vi "Lab Panel V4.84.vi"() -> ()   [LabVIEW 2013] (continued)
                            n2010 = Bundle By Name("Y"=w3276, "t0"=w3271) -> (w3268:waveform(dbl))  [unwired: 1 in]
                            n2011 = Bundle By Name("Y"=w3275, "t0"=w3271) -> (w3267:waveform(dbl))  [unwired: 1 in]
                            n2012 = Bundle By Name("Y"=w3274, "t0"=w3271) -> (w3266:waveform(dbl))  [unwired: 1 in]
                            n2013 = Bundle By Name("Y"=w3273, "t0"=w3271) -> (w3265:waveform(dbl))  [unwired: 1 in]
                            n2014 = Bundle By Name("Y"=w3272, "t0"=w3271) -> (w3264:waveform(dbl))  [unwired: 1 in]
                            n2015 = Build Array(w3270, w3269, w3268, w3267, w3266, w3265, w3264) -> (w3263:waveform(dbl)[])
                            n2016 = TDMS Write(0:w3284, 5:"TEST VALUES", 7:w3255, 9:w3263) -> (4:w3254:refnum<k34>, 6:w3253:string, 15:w3252:errorcluster)  [unwired: 2 in, 1 out]
                            n2017 = TDMS Write(0:w3254, 5:w3253, 7:"TIME", 9:w3250, 11:w3252) -> (15:w3249:errorcluster)  [unwired: 1 in, 3 out]
                            n2018 = local write "data file error"(w3249) -> ()
                          }
                        }
                      }
                    }
                  }
                }
              }
              frame #2 {
                n2019 = case shown="True" w3288 {
                  tunnel: w3292 -> [_ w3297]
                  tunnel: w3291 -> [_ w3296]
                  tunnel: w3290 -> [_ w3294]
                  tunnel: w3289 -> [_ w3293]
                  frame False {
                  }
                  frame True {
                    n2020 = local read "DISP LAB02-1"() -> (w3298:T4)
                    n2021 = local read "SIG LAB02-1"() -> (w3299:T2)
                    n2022 = local read "ON L02-1"() -> (w3295:cluster{"amps":dbl, "volts":dbl, "pf":dbl})
                    n2023 = Unbundle(w3299) -> ("AMPS"=w3305:dbl, "VOLTS"=w3303:dbl, "PF"=w3302:dbl, "Tmp Live"=w3301:dbl, "Tmp Neut"=w3304:dbl)
                    n2024 = Unbundle(w3298) -> ("CYCLE"=w3300:dbl)  [unwired: 2 out]
                    n2025 = stacked-sequence {
                      tunnel: w3305 -> [w3309 w3328]
                      tunnel: w3304 -> [_ w3327]
                      tunnel: w3303 -> [w3308 w3326]
                      tunnel: w3302 -> [w3307 w3325]
                      tunnel: w3301 -> [_ w3324]
                      tunnel: w3300 -> [_ w3323]
                      tunnel: w3297 -> [_ w3322]
                      tunnel: w3296 -> [w3310 _]
                      tunnel: w3295 -> [w3306 w3320]
                      tunnel: w3294 -> [_ w3321]
                      tunnel: w3293 -> [_ w3316]
                      frame #0 {
                        n2026 = case shown="True" w3310 {
                          tunnel: w3309 -> [_ w3315]
                          tunnel: w3308 -> [_ w3314]
                          tunnel: w3307 -> [_ w3313]
                          tunnel: w3306 -> [_ w3311]
                          frame False {
                          }
                          frame True {
                            n2027 = Bundle(cluster=w3311, "amps"=w3315, "volts"=w3314, "pf"=w3313) -> (w3312:cluster{"amps":dbl, "volts":dbl, "pf":dbl})
                            n2028 = local write "ON L02-1"(w3312) -> ()
                          }
                        }
                      }
                      frame #1 {
                        n2029 = Unbundle(w3320) -> ("amps"=w3319:dbl, "volts"=w3318:dbl, "pf"=w3317:dbl)
                        n2030 = case shown="True" w3321 {
                          tunnel: w3328 -> [_ w3360]
                          tunnel: w3327 -> [_ w3367]
                          tunnel: w3326 -> [_ _]
                          tunnel: w3325 -> [_ _]
                          tunnel: w3324 -> [_ w3366]
                          tunnel: w3323 -> [_ w3365]
                          tunnel: w3322 -> [_ w3330]
                          tunnel: w3319 -> [_ w3362]
                          tunnel: w3318 -> [_ w3361]
                          tunnel: w3317 -> [_ w3359]
                          tunnel: w3316 -> [_ w3351]
                          frame False {
                          }
                          frame True {
                            n2031 = local read "TDMS LAB02-1"() -> (w3364:refnum<k34>)
                            n2032 = Build Array(w3361) -> (w3356:dbl[])
                            n2033 = Build Array(w3359) -> (w3355:dbl[])
                            n2034 = Build Array(w3366) -> (w3354:dbl[])
                            n2035 = Build Array(w3367) -> (w3353:dbl[])
                            n2036 = Build Array(w3362) -> (w3358:dbl[])
                            n2037 = Build Array(w3360) -> (w3357:dbl[])
                            n2038 = Build Array(w3365) -> (w3352:dbl[])
                            n2039 = Build Array("AMPS ON", "AMPS OFF", "VOLTS", "PF", "TEMP Live", "TEMP Neut", "CYCLE") -> (w3335:string[])
                            n2040 = Bundle By Name("Y"=w3358, "t0"=w3351) -> (w3350:waveform(dbl))  [unwired: 1 in]
                            n2041 = Bundle By Name("Y"=w3357, "t0"=w3351) -> (w3349:waveform(dbl))  [unwired: 1 in]
                            n2042 = Bundle By Name("Y"=w3356, "t0"=w3351) -> (w3348:waveform(dbl))  [unwired: 1 in]
                            n2043 = Bundle By Name("Y"=w3355, "t0"=w3351) -> (w3347:waveform(dbl))  [unwired: 1 in]
                            n2044 = Bundle By Name("Y"=w3354, "t0"=w3351) -> (w3346:waveform(dbl))  [unwired: 1 in]
                            n2045 = Bundle By Name("Y"=w3353, "t0"=w3351) -> (w3345:waveform(dbl))  [unwired: 1 in]
                            n2046 = Bundle By Name("Y"=w3352, "t0"=w3351) -> (w3344:waveform(dbl))  [unwired: 1 in]
                            n2047 = Build Array(w3350, w3349, w3348, w3347, w3346, w3345, w3344) -> (w3343:waveform(dbl)[])
                            n2048 = TDMS Write(0:w3364, 5:"TEST VALUES", 7:w3335, 9:w3343) -> (4:w3334:refnum<k34>, 6:w3333:string, 15:w3332:errorcluster)  [unwired: 2 in, 1 out]
                            n2049 = TDMS Write(0:w3334, 5:w3333, 7:"TIME", 9:w3330, 11:w3332) -> (15:w3329:errorcluster)  [unwired: 1 in, 3 out]
                            n2050 = local write "data file error"(w3329) -> ()
                          }
                        }
                      }
                    }
                  }
                }
              }
              frame #3 {
                n2051 = case shown="True" w3368 {
                  tunnel: w3372 -> [_ w3377]
                  tunnel: w3371 -> [_ w3376]
                  tunnel: w3370 -> [_ w3374]
                  tunnel: w3369 -> [_ w3373]
                  frame False {
                  }
                  frame True {
                    n2052 = local read "DISP LAB02-2"() -> (w3378:T4)
                    n2053 = local read "SIG LAB02-2"() -> (w3379:T2)
                    n2054 = local read "ON L02-2"() -> (w3375:cluster{"amps":dbl, "volts":dbl, "pf":dbl})
                    n2055 = Unbundle(w3379) -> ("AMPS"=w3385:dbl, "VOLTS"=w3383:dbl, "PF"=w3382:dbl, "Tmp Live"=w3381:dbl, "Tmp Neut"=w3384:dbl)
                    n2056 = Unbundle(w3378) -> ("CYCLE"=w3380:dbl)  [unwired: 2 out]
                    n2057 = stacked-sequence {
                      tunnel: w3385 -> [w3389 w3408]
                      tunnel: w3384 -> [_ w3407]
                      tunnel: w3383 -> [w3388 w3406]
                      tunnel: w3382 -> [w3387 w3405]
                      tunnel: w3381 -> [_ w3404]
                      tunnel: w3380 -> [_ w3403]
                      tunnel: w3377 -> [_ w3402]
                      tunnel: w3376 -> [w3390 _]
                      tunnel: w3375 -> [w3386 w3400]
                      tunnel: w3374 -> [_ w3401]
                      tunnel: w3373 -> [_ w3396]
                      frame #0 {
                        n2058 = case shown="True" w3390 {
                          tunnel: w3389 -> [_ w3395]
                          tunnel: w3388 -> [_ w3394]
                          tunnel: w3387 -> [_ w3393]
                          tunnel: w3386 -> [_ w3391]
                          frame False {
                          }
                          frame True {
                            n2059 = Bundle(cluster=w3391, "amps"=w3395, "volts"=w3394, "pf"=w3393) -> (w3392:cluster{"amps":dbl, "volts":dbl, "pf":dbl})
                            n2060 = local write "ON L02-2"(w3392) -> ()
                          }
                        }
                      }
                      frame #1 {
                        n2061 = Unbundle(w3400) -> ("amps"=w3399:dbl, "volts"=w3398:dbl, "pf"=w3397:dbl)
                        n2062 = case shown="True" w3401 {
                          tunnel: w3408 -> [_ w3440]
                          tunnel: w3407 -> [_ w3447]
                          tunnel: w3406 -> [_ _]
                          tunnel: w3405 -> [_ _]
                          tunnel: w3404 -> [_ w3446]
                          tunnel: w3403 -> [_ w3445]
                          tunnel: w3402 -> [_ w3410]
                          tunnel: w3399 -> [_ w3442]
                          tunnel: w3398 -> [_ w3441]
                          tunnel: w3397 -> [_ w3439]
                          tunnel: w3396 -> [_ w3431]
                          frame False {
                          }
                          frame True {
                            n2063 = local read "TDMS LAB02-2"() -> (w3444:refnum<k34>)
                            n2064 = Build Array(w3441) -> (w3436:dbl[])
                            n2065 = Build Array(w3439) -> (w3435:dbl[])
                            n2066 = Build Array(w3446) -> (w3434:dbl[])
                            n2067 = Build Array(w3447) -> (w3433:dbl[])
                            n2068 = Build Array(w3442) -> (w3438:dbl[])
                            n2069 = Build Array(w3440) -> (w3437:dbl[])
                            n2070 = Build Array(w3445) -> (w3432:dbl[])
                            n2071 = Build Array("AMPS ON", "AMPS OFF", "VOLTS", "PF", "TEMP Live", "TEMP Neut", "CYCLE") -> (w3415:string[])
                            n2072 = Bundle By Name("Y"=w3438, "t0"=w3431) -> (w3430:waveform(dbl))  [unwired: 1 in]
                            n2073 = Bundle By Name("Y"=w3437, "t0"=w3431) -> (w3429:waveform(dbl))  [unwired: 1 in]
                            n2074 = Bundle By Name("Y"=w3436, "t0"=w3431) -> (w3428:waveform(dbl))  [unwired: 1 in]
                            n2075 = Bundle By Name("Y"=w3435, "t0"=w3431) -> (w3427:waveform(dbl))  [unwired: 1 in]
                            n2076 = Bundle By Name("Y"=w3434, "t0"=w3431) -> (w3426:waveform(dbl))  [unwired: 1 in]
                            n2077 = Bundle By Name("Y"=w3433, "t0"=w3431) -> (w3425:waveform(dbl))  [unwired: 1 in]
                            n2078 = Bundle By Name("Y"=w3432, "t0"=w3431) -> (w3424:waveform(dbl))  [unwired: 1 in]
                            n2079 = Build Array(w3430, w3429, w3428, w3427, w3426, w3425, w3424) -> (w3423:waveform(dbl)[])
                            n2080 = TDMS Write(0:w3444, 5:"TEST VALUES", 7:w3415, 9:w3423) -> (4:w3414:refnum<k34>, 6:w3413:string, 15:w3412:errorcluster)  [unwired: 2 in, 1 out]
                            n2081 = TDMS Write(0:w3414, 5:w3413, 7:"TIME", 9:w3410, 11:w3412) -> (15:w3409:errorcluster)  [unwired: 1 in, 3 out]
                            n2082 = local write "data file error"(w3409) -> ()
                          }
                        }
                      }
                    }
                  }
                }
              }
              frame #4 {
                n2083 = case shown="True" w3448 {
                  tunnel: w3452 -> [_ w3457]
                  tunnel: w3451 -> [_ w3456]
                  tunnel: w3450 -> [_ w3454]
                  tunnel: w3449 -> [_ w3453]
                  frame False {
                  }
                  frame True {
                    n2084 = local read "DISP LAB03-1"() -> (w3458:T4)
                    n2085 = local read "SIG LAB03-1"() -> (w3459:T2)
                    n2086 = local read "ON L03-1"() -> (w3455:cluster{"amps":dbl, "volts":dbl, "pf":dbl})
                    n2087 = Unbundle(w3459) -> ("AMPS"=w3465:dbl, "VOLTS"=w3463:dbl, "PF"=w3462:dbl, "Tmp Live"=w3461:dbl, "Tmp Neut"=w3464:dbl)
                    n2088 = Unbundle(w3458) -> ("CYCLE"=w3460:dbl)  [unwired: 2 out]
                    n2089 = stacked-sequence {
                      tunnel: w3465 -> [w3469 w3488]
                      tunnel: w3464 -> [_ w3487]
                      tunnel: w3463 -> [w3468 w3486]
                      tunnel: w3462 -> [w3467 w3485]
                      tunnel: w3461 -> [_ w3484]
                      tunnel: w3460 -> [_ w3483]
                      tunnel: w3457 -> [_ w3482]
                      tunnel: w3456 -> [w3470 _]
                      tunnel: w3455 -> [w3466 w3480]
                      tunnel: w3454 -> [_ w3481]
                      tunnel: w3453 -> [_ w3476]
                      frame #0 {
                        n2090 = case shown="True" w3470 {
                          tunnel: w3469 -> [_ w3475]
                          tunnel: w3468 -> [_ w3474]
                          tunnel: w3467 -> [_ w3473]
                          tunnel: w3466 -> [_ w3471]
                          frame False {
                          }
                          frame True {
                            n2091 = Bundle(cluster=w3471, "amps"=w3475, "volts"=w3474, "pf"=w3473) -> (w3472:cluster{"amps":dbl, "volts":dbl, "pf":dbl})
                            n2092 = local write "ON L03-1"(w3472) -> ()
                          }
                        }
                      }
                      frame #1 {
                        n2093 = Unbundle(w3480) -> ("amps"=w3479:dbl, "volts"=w3478:dbl, "pf"=w3477:dbl)
                        n2094 = case shown="True" w3481 {
                          tunnel: w3488 -> [_ w3520]
                          tunnel: w3487 -> [_ w3527]
                          tunnel: w3486 -> [_ _]
                          tunnel: w3485 -> [_ _]
                          tunnel: w3484 -> [_ w3526]
                          tunnel: w3483 -> [_ w3525]
                          tunnel: w3482 -> [_ w3490]
                          tunnel: w3479 -> [_ w3522]
                          tunnel: w3478 -> [_ w3521]
                          tunnel: w3477 -> [_ w3519]
                          tunnel: w3476 -> [_ w3511]
                          frame False {
                          }
                          frame True {
                            n2095 = local read "TDMS LAB03-1"() -> (w3524:refnum<k34>)
                            n2096 = Build Array(w3521) -> (w3516:dbl[])
                            n2097 = Build Array(w3519) -> (w3515:dbl[])
                            n2098 = Build Array(w3526) -> (w3514:dbl[])
                            n2099 = Build Array(w3527) -> (w3513:dbl[])
                            n2100 = Build Array(w3522) -> (w3518:dbl[])
                            n2101 = Build Array(w3520) -> (w3517:dbl[])
                            n2102 = Build Array(w3525) -> (w3512:dbl[])
                            n2103 = Build Array("AMPS ON", "AMPS OFF", "VOLTS", "PF", "TEMP Live", "TEMP Neut", "CYCLE") -> (w3495:string[])
                            n2104 = Bundle By Name("Y"=w3518, "t0"=w3511) -> (w3510:waveform(dbl))  [unwired: 1 in]
                            n2105 = Bundle By Name("Y"=w3517, "t0"=w3511) -> (w3509:waveform(dbl))  [unwired: 1 in]
                            n2106 = Bundle By Name("Y"=w3516, "t0"=w3511) -> (w3508:waveform(dbl))  [unwired: 1 in]
                            n2107 = Bundle By Name("Y"=w3515, "t0"=w3511) -> (w3507:waveform(dbl))  [unwired: 1 in]
                            n2108 = Bundle By Name("Y"=w3514, "t0"=w3511) -> (w3506:waveform(dbl))  [unwired: 1 in]
                            n2109 = Bundle By Name("Y"=w3513, "t0"=w3511) -> (w3505:waveform(dbl))  [unwired: 1 in]
                            n2110 = Bundle By Name("Y"=w3512, "t0"=w3511) -> (w3504:waveform(dbl))  [unwired: 1 in]
                            n2111 = Build Array(w3510, w3509, w3508, w3507, w3506, w3505, w3504) -> (w3503:waveform(dbl)[])
                            n2112 = TDMS Write(0:w3524, 5:"TEST VALUES", 7:w3495, 9:w3503) -> (4:w3494:refnum<k34>, 6:w3493:string, 15:w3492:errorcluster)  [unwired: 2 in, 1 out]
                            n2113 = TDMS Write(0:w3494, 5:w3493, 7:"TIME", 9:w3490, 11:w3492) -> (15:w3489:errorcluster)  [unwired: 1 in, 3 out]
                            n2114 = local write "data file error"(w3489) -> ()
                          }
                        }
                      }
                    }
                  }
                }
              }
              frame #5 {
                n2115 = case shown="True" w3528 {
                  tunnel: w3532 -> [_ w3537]
                  tunnel: w3531 -> [_ w3536]
                  tunnel: w3530 -> [_ w3534]
                  tunnel: w3529 -> [_ w3533]
                  frame False {
                  }
                  frame True {
                    n2116 = local read "DISP LAB03-2"() -> (w3538:T4)
                    n2117 = local read "SIG LAB03-2"() -> (w3539:T2)
                    n2118 = local read "ON L03-2"() -> (w3535:cluster{"amps":dbl, "volts":dbl, "pf":dbl})
                    n2119 = Unbundle(w3539) -> ("AMPS"=w3545:dbl, "VOLTS"=w3543:dbl, "PF"=w3542:dbl, "Tmp Live"=w3541:dbl, "Tmp Neut"=w3544:dbl)
                    n2120 = Unbundle(w3538) -> ("CYCLE"=w3540:dbl)  [unwired: 2 out]
                    n2121 = stacked-sequence {
                      tunnel: w3545 -> [w3549 w3568]
                      tunnel: w3544 -> [_ w3567]
                      tunnel: w3543 -> [w3548 w3566]
                      tunnel: w3542 -> [w3547 w3565]
                      tunnel: w3541 -> [_ w3564]
                      tunnel: w3540 -> [_ w3563]
                      tunnel: w3537 -> [_ w3562]
                      tunnel: w3536 -> [w3550 _]
                      tunnel: w3535 -> [w3546 w3560]
                      tunnel: w3534 -> [_ w3561]
                      tunnel: w3533 -> [_ w3556]
                      frame #0 {
                        n2122 = case shown="True" w3550 {
                          tunnel: w3549 -> [_ w3555]
                          tunnel: w3548 -> [_ w3554]
                          tunnel: w3547 -> [_ w3553]
                          tunnel: w3546 -> [_ w3551]
                          frame False {
                          }
                          frame True {
                            n2123 = Bundle(cluster=w3551, "amps"=w3555, "volts"=w3554, "pf"=w3553) -> (w3552:cluster{"amps":dbl, "volts":dbl, "pf":dbl})
                            n2124 = local write "ON L03-2"(w3552) -> ()
                          }
                        }
                      }
                      frame #1 {
                        n2125 = Unbundle(w3560) -> ("amps"=w3559:dbl, "volts"=w3558:dbl, "pf"=w3557:dbl)
                        n2126 = case shown="True" w3561 {
                          tunnel: w3568 -> [_ w3600]
                          tunnel: w3567 -> [_ w3607]
                          tunnel: w3566 -> [_ _]
                          tunnel: w3565 -> [_ _]
                          tunnel: w3564 -> [_ w3606]
                          tunnel: w3563 -> [_ w3605]
                          tunnel: w3562 -> [_ w3570]
                          tunnel: w3559 -> [_ w3602]
                          tunnel: w3558 -> [_ w3601]
                          tunnel: w3557 -> [_ w3599]
                          tunnel: w3556 -> [_ w3591]
                          frame False {
                          }
                          frame True {
                            n2127 = local read "TDMS LAB03-2"() -> (w3604:refnum<k34>)
                            n2128 = Build Array(w3601) -> (w3596:dbl[])
                            n2129 = Build Array(w3599) -> (w3595:dbl[])
                            n2130 = Build Array(w3606) -> (w3594:dbl[])
                            n2131 = Build Array(w3607) -> (w3593:dbl[])
                            n2132 = Build Array(w3602) -> (w3598:dbl[])
                            n2133 = Build Array(w3600) -> (w3597:dbl[])
                            n2134 = Build Array(w3605) -> (w3592:dbl[])
                            n2135 = Build Array("AMPS ON", "AMPS OFF", "VOLTS", "PF", "TEMP Live", "TEMP Neut", "CYCLE") -> (w3575:string[])
                            n2136 = Bundle By Name("Y"=w3598, "t0"=w3591) -> (w3590:waveform(dbl))  [unwired: 1 in]
                            n2137 = Bundle By Name("Y"=w3597, "t0"=w3591) -> (w3589:waveform(dbl))  [unwired: 1 in]
                            n2138 = Bundle By Name("Y"=w3596, "t0"=w3591) -> (w3588:waveform(dbl))  [unwired: 1 in]
                            n2139 = Bundle By Name("Y"=w3595, "t0"=w3591) -> (w3587:waveform(dbl))  [unwired: 1 in]
                            n2140 = Bundle By Name("Y"=w3594, "t0"=w3591) -> (w3586:waveform(dbl))  [unwired: 1 in]
                            n2141 = Bundle By Name("Y"=w3593, "t0"=w3591) -> (w3585:waveform(dbl))  [unwired: 1 in]
                            n2142 = Bundle By Name("Y"=w3592, "t0"=w3591) -> (w3584:waveform(dbl))  [unwired: 1 in]
                            n2143 = Build Array(w3590, w3589, w3588, w3587, w3586, w3585, w3584) -> (w3583:waveform(dbl)[])
                            n2144 = TDMS Write(0:w3604, 5:"TEST VALUES", 7:w3575, 9:w3583) -> (4:w3574:refnum<k34>, 6:w3573:string, 15:w3572:errorcluster)  [unwired: 2 in, 1 out]
                            n2145 = TDMS Write(0:w3574, 5:w3573, 7:"TIME", 9:w3570, 11:w3572) -> (15:w3569:errorcluster)  [unwired: 1 in, 3 out]
                            n2146 = local write "data file error"(w3569) -> ()
                          }
                        }
                      }
                    }
                  }
                }
              }
              frame #6 {
                n2147 = case shown="True" w3608 {
                  tunnel: w3612 -> [_ w3617]
                  tunnel: w3611 -> [_ w3616]
                  tunnel: w3610 -> [_ w3614]
                  tunnel: w3609 -> [_ w3613]
                  frame False {
                  }
                  frame True {
                    n2148 = local read "DISP LAB04-1"() -> (w3618:T4)
                    n2149 = local read "SIG LAB04-1"() -> (w3619:T2)
                    n2150 = local read "ON L04-1"() -> (w3615:cluster{"amps":dbl, "volts":dbl, "pf":dbl})
                    n2151 = Unbundle(w3619) -> ("AMPS"=w3625:dbl, "VOLTS"=w3623:dbl, "PF"=w3622:dbl, "Tmp Live"=w3621:dbl, "Tmp Neut"=w3624:dbl)
                    n2152 = Unbundle(w3618) -> ("CYCLE"=w3620:dbl)  [unwired: 2 out]
                    n2153 = stacked-sequence {
                      tunnel: w3625 -> [w3629 w3648]
                      tunnel: w3624 -> [_ w3647]
                      tunnel: w3623 -> [w3628 w3646]
                      tunnel: w3622 -> [w3627 w3645]
                      tunnel: w3621 -> [_ w3644]
                      tunnel: w3620 -> [_ w3643]
                      tunnel: w3617 -> [_ w3642]
                      tunnel: w3616 -> [w3630 _]
                      tunnel: w3615 -> [w3626 w3640]
                      tunnel: w3614 -> [_ w3641]
                      tunnel: w3613 -> [_ w3636]
                      frame #0 {
                        n2154 = case shown="True" w3630 {
                          tunnel: w3629 -> [_ w3635]
                          tunnel: w3628 -> [_ w3634]
                          tunnel: w3627 -> [_ w3633]
                          tunnel: w3626 -> [_ w3631]
                          frame False {
                          }
                          frame True {
                            n2155 = Bundle(cluster=w3631, "amps"=w3635, "volts"=w3634, "pf"=w3633) -> (w3632:cluster{"amps":dbl, "volts":dbl, "pf":dbl})
                            n2156 = local write "ON L04-1"(w3632) -> ()
                          }
                        }
                      }
                      frame #1 {
                        n2157 = Unbundle(w3640) -> ("amps"=w3639:dbl, "volts"=w3638:dbl, "pf"=w3637:dbl)
                        n2158 = case shown="True" w3641 {
                          tunnel: w3648 -> [_ w3680]
                          tunnel: w3647 -> [_ w3687]
                          tunnel: w3646 -> [_ _]
                          tunnel: w3645 -> [_ _]
                          tunnel: w3644 -> [_ w3686]
                          tunnel: w3643 -> [_ w3685]
                          tunnel: w3642 -> [_ w3650]
                          tunnel: w3639 -> [_ w3682]
                          tunnel: w3638 -> [_ w3681]
                          tunnel: w3637 -> [_ w3679]
                          tunnel: w3636 -> [_ w3671]
                          frame False {
                          }
                          frame True {
                            n2159 = local read "TDMS LAB04-1"() -> (w3684:refnum<k34>)
                            n2160 = Build Array(w3681) -> (w3676:dbl[])
                            n2161 = Build Array(w3679) -> (w3675:dbl[])
                            n2162 = Build Array(w3686) -> (w3674:dbl[])
                            n2163 = Build Array(w3687) -> (w3673:dbl[])
                            n2164 = Build Array(w3682) -> (w3678:dbl[])
                            n2165 = Build Array(w3680) -> (w3677:dbl[])
                            n2166 = Build Array(w3685) -> (w3672:dbl[])
                            n2167 = Build Array("AMPS ON", "AMPS OFF", "VOLTS", "PF", "TEMP Live", "TEMP Neut", "CYCLE") -> (w3655:string[])
                            n2168 = Bundle By Name("Y"=w3678, "t0"=w3671) -> (w3670:waveform(dbl))  [unwired: 1 in]
                            n2169 = Bundle By Name("Y"=w3677, "t0"=w3671) -> (w3669:waveform(dbl))  [unwired: 1 in]
                            n2170 = Bundle By Name("Y"=w3676, "t0"=w3671) -> (w3668:waveform(dbl))  [unwired: 1 in]
                            n2171 = Bundle By Name("Y"=w3675, "t0"=w3671) -> (w3667:waveform(dbl))  [unwired: 1 in]
                            n2172 = Bundle By Name("Y"=w3674, "t0"=w3671) -> (w3666:waveform(dbl))  [unwired: 1 in]
                            n2173 = Bundle By Name("Y"=w3673, "t0"=w3671) -> (w3665:waveform(dbl))  [unwired: 1 in]
                            n2174 = Bundle By Name("Y"=w3672, "t0"=w3671) -> (w3664:waveform(dbl))  [unwired: 1 in]
                            n2175 = Build Array(w3670, w3669, w3668, w3667, w3666, w3665, w3664) -> (w3663:waveform(dbl)[])
                            n2176 = TDMS Write(0:w3684, 5:"TEST VALUES", 7:w3655, 9:w3663) -> (4:w3654:refnum<k34>, 6:w3653:string, 15:w3652:errorcluster)  [unwired: 2 in, 1 out]
                            n2177 = TDMS Write(0:w3654, 5:w3653, 7:"TIME", 9:w3650, 11:w3652) -> (15:w3649:errorcluster)  [unwired: 1 in, 3 out]
                            n2178 = local write "data file error"(w3649) -> ()
                          }
                        }
                      }
                    }
                  }
                }
              }
              frame #7 {
                n2179 = case shown="True" w3688 {
                  tunnel: w3692 -> [_ w3697]
                  tunnel: w3691 -> [_ w3696]
                  tunnel: w3690 -> [_ w3694]
                  tunnel: w3689 -> [_ w3693]
                  frame False {
                  }
                  frame True {
                    n2180 = local read "DISP LAB04-2"() -> (w3698:T4)
                    n2181 = local read "SIG LAB04-2"() -> (w3699:T2)
                    n2182 = local read "ON L04-2"() -> (w3695:cluster{"amps":dbl, "volts":dbl, "pf":dbl})
                    n2183 = Unbundle(w3699) -> ("AMPS"=w3705:dbl, "VOLTS"=w3703:dbl, "PF"=w3702:dbl, "Tmp Live"=w3701:dbl, "Tmp Neut"=w3704:dbl)
                    n2184 = Unbundle(w3698) -> ("CYCLE"=w3700:dbl)  [unwired: 2 out]
                    n2185 = stacked-sequence {
                      tunnel: w3705 -> [w3709 w3728]
                      tunnel: w3704 -> [_ w3727]
                      tunnel: w3703 -> [w3708 w3726]
                      tunnel: w3702 -> [w3707 w3725]
                      tunnel: w3701 -> [_ w3724]
                      tunnel: w3700 -> [_ w3723]
                      tunnel: w3697 -> [_ w3722]
                      tunnel: w3696 -> [w3710 _]
                      tunnel: w3695 -> [w3706 w3720]
                      tunnel: w3694 -> [_ w3721]
                      tunnel: w3693 -> [_ w3716]
                      frame #0 {
                        n2186 = case shown="True" w3710 {
                          tunnel: w3709 -> [_ w3715]
                          tunnel: w3708 -> [_ w3714]
                          tunnel: w3707 -> [_ w3713]
                          tunnel: w3706 -> [_ w3711]
                          frame False {
                          }
                          frame True {
                            n2187 = Bundle(cluster=w3711, "amps"=w3715, "volts"=w3714, "pf"=w3713) -> (w3712:cluster{"amps":dbl, "volts":dbl, "pf":dbl})
                            n2188 = local write "ON L04-2"(w3712) -> ()
                          }
                        }
                      }
                      frame #1 {
                        n2189 = Unbundle(w3720) -> ("amps"=w3719:dbl, "volts"=w3718:dbl, "pf"=w3717:dbl)
                        n2190 = case shown="True" w3721 {
                          tunnel: w3728 -> [_ w3760]
                          tunnel: w3727 -> [_ w3767]
                          tunnel: w3726 -> [_ _]
                          tunnel: w3725 -> [_ _]
                          tunnel: w3724 -> [_ w3766]
                          tunnel: w3723 -> [_ w3765]
                          tunnel: w3722 -> [_ w3730]
                          tunnel: w3719 -> [_ w3762]
                          tunnel: w3718 -> [_ w3761]
                          tunnel: w3717 -> [_ w3759]
                          tunnel: w3716 -> [_ w3751]
                          frame False {
                          }
                          frame True {
                            n2191 = local read "TDMS LAB04-2"() -> (w3764:refnum<k34>)
                            n2192 = Build Array(w3761) -> (w3756:dbl[])
                            n2193 = Build Array(w3759) -> (w3755:dbl[])
                            n2194 = Build Array(w3766) -> (w3754:dbl[])
                            n2195 = Build Array(w3767) -> (w3753:dbl[])
                            n2196 = Build Array(w3762) -> (w3758:dbl[])
                            n2197 = Build Array(w3760) -> (w3757:dbl[])
                            n2198 = Build Array(w3765) -> (w3752:dbl[])
                            n2199 = Build Array("AMPS ON", "AMPS OFF", "VOLTS", "PF", "TEMP Live", "TEMP Neut", "CYCLE") -> (w3735:string[])
                            n2200 = Bundle By Name("Y"=w3758, "t0"=w3751) -> (w3750:waveform(dbl))  [unwired: 1 in]
                            n2201 = Bundle By Name("Y"=w3757, "t0"=w3751) -> (w3749:waveform(dbl))  [unwired: 1 in]
                            n2202 = Bundle By Name("Y"=w3756, "t0"=w3751) -> (w3748:waveform(dbl))  [unwired: 1 in]
                            n2203 = Bundle By Name("Y"=w3755, "t0"=w3751) -> (w3747:waveform(dbl))  [unwired: 1 in]
                            n2204 = Bundle By Name("Y"=w3754, "t0"=w3751) -> (w3746:waveform(dbl))  [unwired: 1 in]
                            n2205 = Bundle By Name("Y"=w3753, "t0"=w3751) -> (w3745:waveform(dbl))  [unwired: 1 in]
                            n2206 = Bundle By Name("Y"=w3752, "t0"=w3751) -> (w3744:waveform(dbl))  [unwired: 1 in]
                            n2207 = Build Array(w3750, w3749, w3748, w3747, w3746, w3745, w3744) -> (w3743:waveform(dbl)[])
                            n2208 = TDMS Write(0:w3764, 5:"TEST VALUES", 7:w3735, 9:w3743) -> (4:w3734:refnum<k34>, 6:w3733:string, 15:w3732:errorcluster)  [unwired: 2 in, 1 out]
                            n2209 = TDMS Write(0:w3734, 5:w3733, 7:"TIME", 9:w3730, 11:w3732) -> (15:w3729:errorcluster)  [unwired: 1 in, 3 out]
                            n2210 = local write "data file error"(w3729) -> ()
                          }
                        }
                      }
                    }
                  }
                }
              }
              frame #8 {
                n2211 = case shown="True" w3768 {
                  tunnel: w3772 -> [_ w3777]
                  tunnel: w3771 -> [_ w3776]
                  tunnel: w3770 -> [_ w3774]
                  tunnel: w3769 -> [_ w3773]
                  frame False {
                  }
                  frame True {
                    n2212 = local read "DISP LAB05-1"() -> (w3778:T4)
                    n2213 = local read "SIG LAB05-1"() -> (w3779:T2)
                    n2214 = local read "ON L05-1"() -> (w3775:cluster{"amps":dbl, "volts":dbl, "pf":dbl})
                    n2215 = Unbundle(w3779) -> ("AMPS"=w3785:dbl, "VOLTS"=w3783:dbl, "PF"=w3782:dbl, "Tmp Live"=w3781:dbl, "Tmp Neut"=w3784:dbl)
                    n2216 = Unbundle(w3778) -> ("CYCLE"=w3780:dbl)  [unwired: 2 out]
                    n2217 = stacked-sequence {
                      tunnel: w3785 -> [w3789 w3808]
                      tunnel: w3784 -> [_ w3807]
                      tunnel: w3783 -> [w3788 w3806]
                      tunnel: w3782 -> [w3787 w3805]
                      tunnel: w3781 -> [_ w3804]
                      tunnel: w3780 -> [_ w3803]
                      tunnel: w3777 -> [_ w3802]
                      tunnel: w3776 -> [w3790 _]
                      tunnel: w3775 -> [w3786 w3800]
                      tunnel: w3774 -> [_ w3801]
                      tunnel: w3773 -> [_ w3796]
                      frame #0 {
                        n2218 = case shown="True" w3790 {
                          tunnel: w3789 -> [_ w3795]
                          tunnel: w3788 -> [_ w3794]
                          tunnel: w3787 -> [_ w3793]
                          tunnel: w3786 -> [_ w3791]
                          frame False {
                          }
                          frame True {
                            n2219 = Bundle(cluster=w3791, "amps"=w3795, "volts"=w3794, "pf"=w3793) -> (w3792:cluster{"amps":dbl, "volts":dbl, "pf":dbl})
                            n2220 = local write "ON L05-1"(w3792) -> ()
                          }
                        }
                      }
                      frame #1 {
                        n2221 = Unbundle(w3800) -> ("amps"=w3799:dbl, "volts"=w3798:dbl, "pf"=w3797:dbl)
                        n2222 = case shown="True" w3801 {
                          tunnel: w3808 -> [_ w3840]
                          tunnel: w3807 -> [_ w3847]
                          tunnel: w3806 -> [_ _]
                          tunnel: w3805 -> [_ _]
                          tunnel: w3804 -> [_ w3846]
                          tunnel: w3803 -> [_ w3845]
                          tunnel: w3802 -> [_ w3810]
                          tunnel: w3799 -> [_ w3842]
                          tunnel: w3798 -> [_ w3841]
                          tunnel: w3797 -> [_ w3839]
                          tunnel: w3796 -> [_ w3831]
                          frame False {
                          }
                          frame True {
                            n2223 = local read "TDMS LAB05-1"() -> (w3844:refnum<k34>)
                            n2224 = Build Array(w3841) -> (w3836:dbl[])
                            n2225 = Build Array(w3839) -> (w3835:dbl[])
                            n2226 = Build Array(w3846) -> (w3834:dbl[])
                            n2227 = Build Array(w3847) -> (w3833:dbl[])
                            n2228 = Build Array(w3842) -> (w3838:dbl[])
                            n2229 = Build Array(w3840) -> (w3837:dbl[])
                            n2230 = Build Array(w3845) -> (w3832:dbl[])
                            n2231 = Build Array("AMPS ON", "AMPS OFF", "VOLTS", "PF", "TEMP Live", "TEMP Neut", "CYCLE") -> (w3815:string[])
                            n2232 = Bundle By Name("Y"=w3838, "t0"=w3831) -> (w3830:waveform(dbl))  [unwired: 1 in]
                            n2233 = Bundle By Name("Y"=w3837, "t0"=w3831) -> (w3829:waveform(dbl))  [unwired: 1 in]
                            n2234 = Bundle By Name("Y"=w3836, "t0"=w3831) -> (w3828:waveform(dbl))  [unwired: 1 in]
                            n2235 = Bundle By Name("Y"=w3835, "t0"=w3831) -> (w3827:waveform(dbl))  [unwired: 1 in]
                            n2236 = Bundle By Name("Y"=w3834, "t0"=w3831) -> (w3826:waveform(dbl))  [unwired: 1 in]
                            n2237 = Bundle By Name("Y"=w3833, "t0"=w3831) -> (w3825:waveform(dbl))  [unwired: 1 in]
                            n2238 = Bundle By Name("Y"=w3832, "t0"=w3831) -> (w3824:waveform(dbl))  [unwired: 1 in]
                            n2239 = Build Array(w3830, w3829, w3828, w3827, w3826, w3825, w3824) -> (w3823:waveform(dbl)[])
                            n2240 = TDMS Write(0:w3844, 5:"TEST VALUES", 7:w3815, 9:w3823) -> (4:w3814:refnum<k34>, 6:w3813:string, 15:w3812:errorcluster)  [unwired: 2 in, 1 out]
                            n2241 = TDMS Write(0:w3814, 5:w3813, 7:"TIME", 9:w3810, 11:w3812) -> (15:w3809:errorcluster)  [unwired: 1 in, 3 out]
                            n2242 = local write "data file error"(w3809) -> ()
                          }
                        }
                      }
                    }
                  }
                }
              }
              frame #9 {
                n2243 = case shown="True" w3848 {
                  tunnel: w3852 -> [_ w3857]
                  tunnel: w3851 -> [_ w3856]
                  tunnel: w3850 -> [_ w3854]
                  tunnel: w3849 -> [_ w3853]
                  frame False {
                  }
                  frame True {
                    n2244 = local read "DISP LAB05-2"() -> (w3858:T4)
                    n2245 = local read "SIG LAB05-2"() -> (w3859:T2)
                    n2246 = local read "ON L05-2"() -> (w3855:cluster{"amps":dbl, "volts":dbl, "pf":dbl})
                    n2247 = Unbundle(w3859) -> ("AMPS"=w3865:dbl, "VOLTS"=w3863:dbl, "PF"=w3862:dbl, "Tmp Live"=w3861:dbl, "Tmp Neut"=w3864:dbl)
                    n2248 = Unbundle(w3858) -> ("CYCLE"=w3860:dbl)  [unwired: 2 out]
                    n2249 = stacked-sequence {
                      tunnel: w3865 -> [w3869 w3888]
                      tunnel: w3864 -> [_ w3887]
                      tunnel: w3863 -> [w3868 w3886]
                      tunnel: w3862 -> [w3867 w3885]
                      tunnel: w3861 -> [_ w3884]
                      tunnel: w3860 -> [_ w3883]
                      tunnel: w3857 -> [_ w3882]
                      tunnel: w3856 -> [w3870 _]
                      tunnel: w3855 -> [w3866 w3880]
                      tunnel: w3854 -> [_ w3881]
                      tunnel: w3853 -> [_ w3876]
                      frame #0 {
                        n2250 = case shown="True" w3870 {
                          tunnel: w3869 -> [_ w3875]
                          tunnel: w3868 -> [_ w3874]
                          tunnel: w3867 -> [_ w3873]
                          tunnel: w3866 -> [_ w3871]
                          frame False {
                          }
                          frame True {
                            n2251 = Bundle(cluster=w3871, "amps"=w3875, "volts"=w3874, "pf"=w3873) -> (w3872:cluster{"amps":dbl, "volts":dbl, "pf":dbl})
                            n2252 = local write "ON L05-2"(w3872) -> ()
                          }
                        }
                      }
                      frame #1 {
                        n2253 = Unbundle(w3880) -> ("amps"=w3879:dbl, "volts"=w3878:dbl, "pf"=w3877:dbl)
                        n2254 = case shown="True" w3881 {
                          tunnel: w3888 -> [_ w3920]
                          tunnel: w3887 -> [_ w3927]
                          tunnel: w3886 -> [_ _]
                          tunnel: w3885 -> [_ _]
                          tunnel: w3884 -> [_ w3926]
                          tunnel: w3883 -> [_ w3925]
                          tunnel: w3882 -> [_ w3890]
                          tunnel: w3879 -> [_ w3922]
                          tunnel: w3878 -> [_ w3921]
                          tunnel: w3877 -> [_ w3919]
                          tunnel: w3876 -> [_ w3911]
                          frame False {
                          }
                          frame True {
                            n2255 = local read "TDMS LAB05-2"() -> (w3924:refnum<k34>)
                            n2256 = Build Array(w3921) -> (w3916:dbl[])
                            n2257 = Build Array(w3919) -> (w3915:dbl[])
                            n2258 = Build Array(w3926) -> (w3914:dbl[])
                            n2259 = Build Array(w3927) -> (w3913:dbl[])
                            n2260 = Build Array(w3922) -> (w3918:dbl[])
                            n2261 = Build Array(w3920) -> (w3917:dbl[])
                            n2262 = Build Array(w3925) -> (w3912:dbl[])
                            n2263 = Build Array("AMPS ON", "AMPS OFF", "VOLTS", "PF", "TEMP Live", "TEMP Neut", "CYCLE") -> (w3895:string[])
                            n2264 = Bundle By Name("Y"=w3918, "t0"=w3911) -> (w3910:waveform(dbl))  [unwired: 1 in]
                            n2265 = Bundle By Name("Y"=w3917, "t0"=w3911) -> (w3909:waveform(dbl))  [unwired: 1 in]
                            n2266 = Bundle By Name("Y"=w3916, "t0"=w3911) -> (w3908:waveform(dbl))  [unwired: 1 in]
                            n2267 = Bundle By Name("Y"=w3915, "t0"=w3911) -> (w3907:waveform(dbl))  [unwired: 1 in]
                            n2268 = Bundle By Name("Y"=w3914, "t0"=w3911) -> (w3906:waveform(dbl))  [unwired: 1 in]
                            n2269 = Bundle By Name("Y"=w3913, "t0"=w3911) -> (w3905:waveform(dbl))  [unwired: 1 in]
                            n2270 = Bundle By Name("Y"=w3912, "t0"=w3911) -> (w3904:waveform(dbl))  [unwired: 1 in]
                            n2271 = Build Array(w3910, w3909, w3908, w3907, w3906, w3905, w3904) -> (w3903:waveform(dbl)[])
                            n2272 = TDMS Write(0:w3924, 5:"TEST VALUES", 7:w3895, 9:w3903) -> (4:w3894:refnum<k34>, 6:w3893:string, 15:w3892:errorcluster)  [unwired: 2 in, 1 out]
                            n2273 = TDMS Write(0:w3894, 5:w3893, 7:"TIME", 9:w3890, 11:w3892) -> (15:w3889:errorcluster)  [unwired: 1 in, 3 out]
                            n2274 = local write "data file error"(w3889) -> ()
                          }
                        }
                      }
                    }
                  }
                }
              }
            }
          }
          frame #13 {
            # "display test values on chart"
            n2275 = disable-structure shown="Disabled" {
              frame Disabled {
                n2276 = case shown="\"ON CYCLE\", Default" "Select  Cycle" {
                  tunnel: [1 _] -> _
                  frame "ON CYCLE", Default {
                  }
                  frame "OFF CYCLE" {
                  }
                }
              }
              frame Enabled {
              }
            }
            n2277 = local read "jig cycle"() -> (w3932:dbl)
            n2278 = local read "on loops"() -> (w3934:dbl)
            n2279 = Add(x=w3934, y=2) -> (x+y=w3931:dbl)
            n2280 = Equal?(x=w3932, y=1) -> (x = y?=w3930:bool)
            n2281 = Equal?(x=w3932, y=w3931) -> (x = y?=w3929:bool)
            n2282 = Or(x=w3930, y=w3929) -> (x .or. y?=w3928:bool)
            "graph flag" <- w3928
            n2283 = global write "Global display 3.vi" "graph flag"(w3928) -> ()
            n2284 = case shown="True" w3928 {
              frame False {
              }
              frame True {
                n2285 = local read "SIG LAB05-1"() -> (w3979:T2)
                n2286 = local read "SIG LAB04-2"() -> (w3980:T2)
                n2287 = local read "SIG LAB05-2"() -> (w3978:T2)
                n2288 = local read "SIG LAB04-1"() -> (w3981:T2)
                n2289 = local read "SIG LAB03-1"() -> (w3983:T2)
                n2290 = local read "SIG LAB03-2"() -> (w3982:T2)
                n2291 = local read "SIG LAB01-1"() -> (w3987:T2)
                n2292 = local read "SIG LAB02-2"() -> (w3984:T2)
                n2293 = local read "SIG LAB02-1"() -> (w3985:T2)
                n2294 = local read "SIG LAB01-2"() -> (w3986:T2)
                n2295 = Unbundle(w3980) -> ("AMPS"=w3970:dbl, "VOLTS"=w3960:dbl, "Tmp Live"=w3950:dbl, "Tmp Neut"=w3940:dbl)  [unwired: 1 out]
                n2296 = Unbundle(w3979) -> ("AMPS"=w3969:dbl, "VOLTS"=w3959:dbl, "Tmp Live"=w3949:dbl, "Tmp Neut"=w3939:dbl)  [unwired: 1 out]
                n2297 = Unbundle(w3978) -> ("AMPS"=w3968:dbl, "VOLTS"=w3958:dbl, "Tmp Live"=w3948:dbl, "Tmp Neut"=w3938:dbl)  [unwired: 1 out]
                n2298 = Unbundle(w3981) -> ("AMPS"=w3971:dbl, "VOLTS"=w3961:dbl, "Tmp Live"=w3951:dbl, "Tmp Neut"=w3941:dbl)  [unwired: 1 out]
                n2299 = Unbundle(w3982) -> ("AMPS"=w3972:dbl, "VOLTS"=w3962:dbl, "Tmp Live"=w3952:dbl, "Tmp Neut"=w3942:dbl)  [unwired: 1 out]
                n2300 = Unbundle(w3983) -> ("AMPS"=w3973:dbl, "VOLTS"=w3963:dbl, "Tmp Live"=w3953:dbl, "Tmp Neut"=w3943:dbl)  [unwired: 1 out]
                n2301 = Unbundle(w3984) -> ("AMPS"=w3974:dbl, "VOLTS"=w3964:dbl, "Tmp Live"=w3954:dbl, "Tmp Neut"=w3944:dbl)  [unwired: 1 out]
                n2302 = Unbundle(w3985) -> ("AMPS"=w3975:dbl, "VOLTS"=w3965:dbl, "Tmp Live"=w3955:dbl, "Tmp Neut"=w3945:dbl)  [unwired: 1 out]
                n2303 = Unbundle(w3987) -> ("AMPS"=w3977:dbl, "VOLTS"=w3967:dbl, "Tmp Live"=w3957:dbl, "Tmp Neut"=w3947:dbl)  [unwired: 1 out]
                n2304 = Unbundle(w3986) -> ("AMPS"=w3976:dbl, "VOLTS"=w3966:dbl, "Tmp Live"=w3956:dbl, "Tmp Neut"=w3946:dbl)  [unwired: 1 out]
                n2305 = stacked-sequence {
                  tunnel: w3977 -> [w3998 _ _ _ _]
                  tunnel: w3976 -> [w3997 _ _ _ _]
                  tunnel: w3975 -> [w3996 _ _ _ _]
                  tunnel: w3974 -> [w3995 _ _ _ _]
                  tunnel: w3973 -> [w3994 _ _ _ _]
                  tunnel: w3972 -> [w3993 _ _ _ _]
                  tunnel: w3971 -> [w3992 _ _ _ _]
                  tunnel: w3970 -> [w3991 _ _ _ _]
                  tunnel: w3969 -> [w3990 _ _ _ _]
                  tunnel: w3968 -> [w3989 _ _ _ _]
                  tunnel: w3967 -> [_ w4009 _ _ _]
                  tunnel: w3966 -> [_ w4008 _ _ _]
                  tunnel: w3965 -> [_ w4007 _ _ _]
                  tunnel: w3964 -> [_ w4006 _ _ _]
                  tunnel: w3963 -> [_ w4005 _ _ _]
                  tunnel: w3962 -> [_ w4004 _ _ _]
                  tunnel: w3961 -> [_ w4003 _ _ _]
                  tunnel: w3960 -> [_ w4002 _ _ _]
                  tunnel: w3959 -> [_ w4001 _ _ _]
                  tunnel: w3958 -> [_ w4000 _ _ _]
                  tunnel: w3957 -> [_ _ w4020 _ _]
                  tunnel: w3956 -> [_ _ w4019 _ _]
                  tunnel: w3955 -> [_ _ w4018 _ _]
                  tunnel: w3954 -> [_ _ w4017 _ _]
                  tunnel: w3953 -> [_ _ w4016 _ _]
                  tunnel: w3952 -> [_ _ w4015 _ _]
                  tunnel: w3951 -> [_ _ w4014 _ _]
                  tunnel: w3950 -> [_ _ w4013 _ _]
                  tunnel: w3949 -> [_ _ w4012 _ _]
                  tunnel: w3948 -> [_ _ w4011 _ _]
                  tunnel: w3947 -> [_ _ _ w4031 _]
                  tunnel: w3946 -> [_ _ _ w4030 _]
                  tunnel: w3945 -> [_ _ _ w4029 _]
                  tunnel: w3944 -> [_ _ _ w4028 _]
                  tunnel: w3943 -> [_ _ _ w4027 _]
                  tunnel: w3942 -> [_ _ _ w4026 _]
                  tunnel: w3941 -> [_ _ _ w4025 _]
                  tunnel: w3940 -> [_ _ _ w4024 _]
                  tunnel: w3939 -> [_ _ _ w4023 _]
                  tunnel: w3938 -> [_ _ _ w4022 _]
                  frame #0 {
                    n2306 = Merge Signals(w3998, w3997, w3996, w3995, w3994, w3993, w3992, w3991, w3990, w3989) -> (→"TEST AMPS CHART":dynamicdata)
                  }
                  frame #1 {
                    n2307 = Merge Signals(w4009, w4008, w4007, w4006, w4005, w4004, w4003, w4002, w4001, w4000) -> (→"TEST VOLTS CHART":dynamicdata)
                  }
                  frame #2 {
                    n2308 = Merge Signals(w4020, w4019, w4018, w4017, w4016, w4015, w4014, w4013, w4012, w4011) -> (→"TEMPERATURE (L) CHART":dynamicdata)
